vi "Math.vi"(8 "error in (no error)":errorcluster, 11 "Modulo a obtener":T1=enum."Error") -> (0 "error out":errorcluster)   [LabVIEW 2018]
uses:
  Comunes/Controles/Lista Modulos.ctl
  Comunes/Controles/FGV Opciones.ctl
  Comunes/Comunicacion/Mensajes.lvlib
types:
  T1 = typedef "Lista Modulos.ctl" = enum16{"Math", "Error", "Front", "Database", "Nuevos items"}
  T2 = typedef "FGV Opciones.ctl" = enum16{"Get", "Create", "Destroy"}
  T3 = enum32{"Invalid", "Standard", "Closed", "Hidden", "Minimized", "Maximized"}
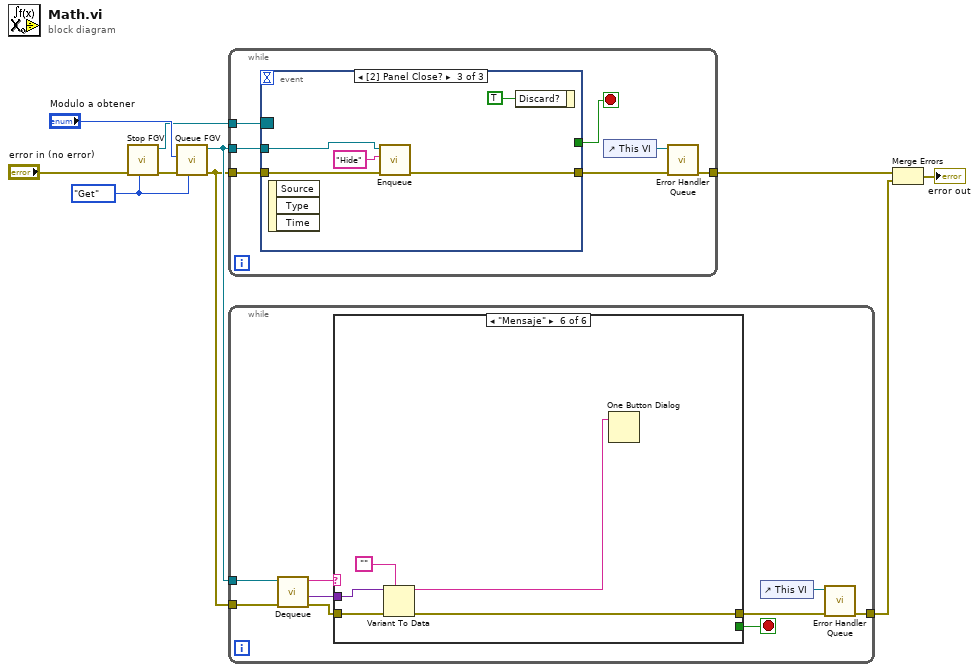
[diagram p0: block diagram]
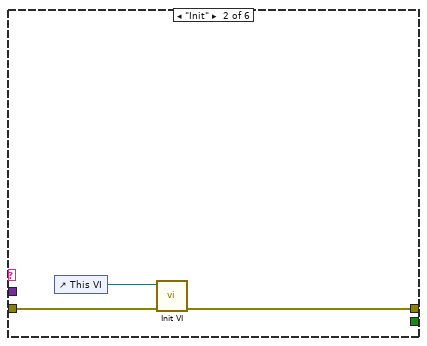
[diagram p3: hidden frame]
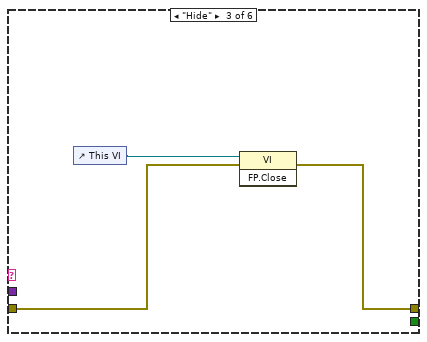
[diagram p4: hidden frame]
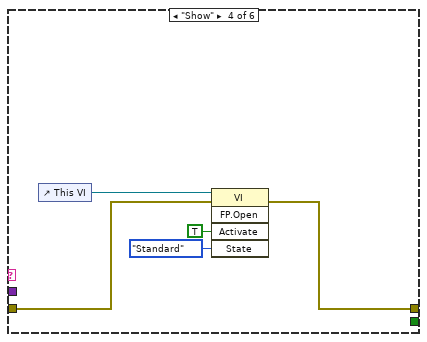
[diagram p5: hidden frame]
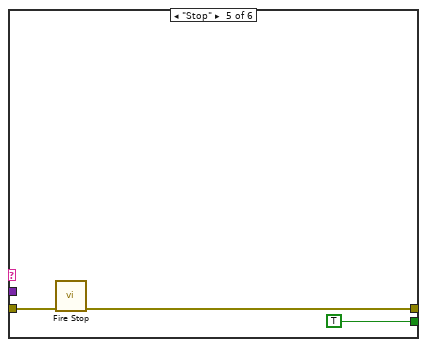
[diagram p6: hidden frame]
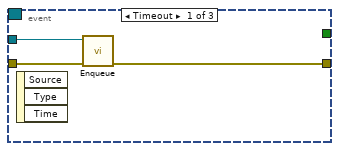
[diagram p7: hidden frame]
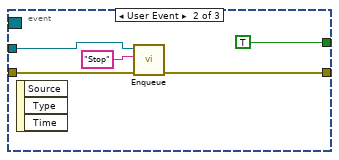
[diagram p8: hidden frame]
diagram:
  w1 = FGV_Opciones."Get" ("Enum")
  n1 = call "Stop FGV.vi"("Enum"=w1, "error in (no error)"="error in (no error)") -> ("error out"=w2:errorcluster, "Event Registration Refnum"=w4:refnum<event-registration>)  [unwired: 7 in, 1 out]
  n2 = call "Queue FGV.vi"("Enum"=w1, "error in (no error)"=w2, "Modulo a obtener"="Modulo a obtener") -> ("error out"=w8:errorcluster, "Queue Ref"=w9:refnum<queue>)  [unwired: 7 in]
  n3 = while {
    tunnel: w9 -> [w17]
    tunnel: w8 -> [w16]
    tunnel: [w14] -> w7
    tunnel: w4 -> [w12]
    stop <- w11 stop-if-true
    n4 = event shown="[2] Panel Close?" {
      selector: w12 -> [_ _ _]
      dyn-events: _ -> [_ _ _]
      timeout: _ -> [_ _ _]
      tunnel: w17 -> [w20 w23 w29]
      tunnel: w16 -> [w19 w24 w28]
      tunnel: [w18 w21 w26] -> w13
      tunnel: [_ TRUE _] -> w11
      event Timeout {
        n5 = event-data() -> ()  [unwired: 1 in, 3 out]
        n6 = call "Enqueue.vi"("error in (no error)"=w19, "Queue in"=w20) -> ("error out"=w18:errorcluster)  [unwired: 9 in]
      }
      event User Event {
        n7 = event-data() -> ()  [unwired: 1 in, 3 out]
        n8 = call "Enqueue.vi"("error in (no error)"=w24, "Mensaje"="Stop", "Queue in"=w23) -> ("error out"=w21:errorcluster)  [unwired: 8 in]
      }
      event Panel Close? {
        n9 = event-data() -> ()  [unwired: 1 in, 3 out]
        n10 = call "Enqueue.vi"("error in (no error)"=w28, "Mensaje"="Hide", "Queue in"=w29) -> ("error out"=w26:errorcluster)  [unwired: 8 in]
        n11 = event-data("Discard?"=TRUE) -> ()  [unwired: 1 in, 1 out]
      }
    }
    n12 = control-ref of="This VI"() -> (w15:refnum<vi>)
    n13 = call "Error Handler Queue.vi"("error in (no error)"=w13, "VI Refnum"=w15) -> ("error out"=w14:errorcluster)  [unwired: 9 in]
  }
  n14 = while {
    tunnel: w9 -> [w39]
    tunnel: w8 -> [w38]
    tunnel: [w32] -> w6
    stop <- w31 stop-if-true
    n15 = call "Dequeue.vi"("error in (no error)"=w38, "Queue in"=w39) -> ("error out"=w34:errorcluster, "Dato"=w36:variant, "Mensaje"=w37:string)  [unwired: 7 in]
    n16 = case shown="\"Mensaje\"" w37 {
      tunnel: w36 -> [_ _ _ _ _ w58]
      tunnel: w34 -> [w40 w43 w45 w48 w54 w59]
      tunnel: [w40 w42 w44 w47 w52 w56] -> w33
      tunnel: [_ _ _ _ TRUE _] -> w31
      frame "False", Default {
      }
      frame "Init" {
        n17 = control-ref of="This VI"() -> (w41:refnum<vi>)
        n18 = call "Init VI.vi"("error in (no error)"=w43, "VI in"=w41) -> ("error out"=w42:errorcluster)  [unwired: 9 in]
      }
      frame "Hide" {
        n19 = control-ref of="This VI"() -> (w46:refnum<vi>)
        n20 = invoke class="VI" method="FP.Close"(reference=w46, error in=w45) -> (error out=w44:errorcluster)  [unwired: 1 in, 2 out]
      }
      frame "Show" {
        n21 = control-ref of="This VI"() -> (w49:refnum<vi>)
        n22 = invoke class="VI" method="FP.Open"(reference=w49, error in=w48, "Activate"=TRUE ("Activate?"), "State"=T3."Standard") -> (error out=w47:errorcluster)  [unwired: 1 in, 4 out]
      }
      frame "Stop" {
        n23 = call "Fire Stop.vi"("error in (no error)"=w54) -> ("error out"=w52:errorcluster)  [unwired: 10 in]
      }
      frame "Mensaje" {
        n24 = Variant To Data(error in=w59, type="", Variant=w58) -> (data=w55:string, error out=w56:errorcluster)
        n25 = One Button Dialog(message=w55) -> ()  [unwired: 1 in, 1 out]
      }
    }
    n26 = control-ref of="This VI"() -> (w35:refnum<vi>)
    n27 = call "Error Handler Queue.vi"("error in (no error)"=w33, "VI Refnum"=w35) -> ("error out"=w32:errorcluster)  [unwired: 9 in]
  }
  n28 = Merge Errors(w7, w6) -> (→"error out":errorcluster)
